vi "Send Ping N Times.vi"(7 "Message Priority (Normal)":T2=enum."Normal", 8 "error in (no error)":errorcluster, 10 "Ping Test":T1, 11 "Message Enqueuer":refnum<class "Message Enqueuer.lvclass">) -> (0 "error out":errorcluster, 3 "Message Enqueuer out":refnum<class "Message Enqueuer.lvclass">)   [LabVIEW 2017, in "Network Test.lvlib" / "Ping N Times Msg.lvclass"]
doc: "This VI sends the message to an actor."
uses:
  Ping N Times Msg.lvclass
  <vilib>/ActorFramework/Message Enqueuer/Message Enqueuer.lvclass
  <vilib>/ActorFramework/Message Enqueuer/Message Priority.ctl
  Network Test/Ping Test Configuration.ctl
  C:/Program Files (x86)/National Instruments/LabVIEW 2017/vi.lib/ActorFramework/Message/Message.lvclass
  Ping N Times Msg.lvclass/Ping N Times Msg.ctl
  <vilib>/ActorFramework/Message Enqueuer/Message Enqueuer.lvclass/Message Enqueuer.ctl
  <vilib>/ActorFramework/Message Priority Queue/Priority Enqueue.vi
  Network Test/Network Test.lvlib
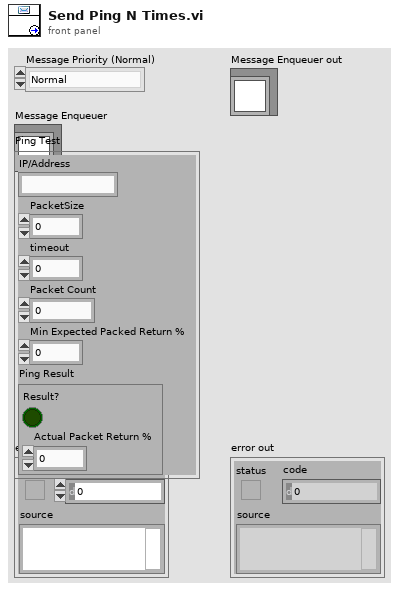
[diagram p1: front panel]
types:
  T1 = typedef "Network Test.lvlib/Ping Test Configuration.ctl" = cluster{"IP/Address":string, "PacketSize":i32, "timeout":i32, "Packet Count":i32, "Min Expected Packed Return %":dbl, "Ping Result":cluster{"Result?":bool, "Actual Packet Return %":dbl}}
  T2 = typedef "Actor Framework.lvlib/Message Enqueuer.lvclass/Message Priority.ctl" = enum16{"Low", "Normal", "High"}
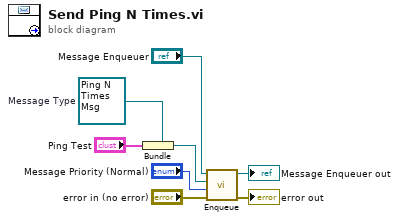
[diagram p0: block diagram]
diagram:
  w2 = refnum<class "Ping N Times Msg.lvclass"> refnum  # Message Type
  n1 = Bundle(cluster=w2, "Ping Test") -> (w3:refnum<class "Ping N Times Msg.lvclass">)
  n2 = call <vilib>:"Enqueue.vi"("error in (no error)"="error in (no error)", "Message Priority (Normal)"="Message Priority (Normal)", "Message"=w3, "Message Enqueuer in"="Message Enqueuer") -> ("error out"=→"error out":errorcluster, "Message Enqueuer out"=→"Message Enqueuer out":refnum<class "Message Enqueuer.lvclass">)  [unwired: 6 in]
